vi "03 LV - Staged create-verify-staged update-archive.vi"   [LabVIEW 2020]
uses:
  client/Client/Client.lvclass
  client/AssetCreateStaging/AssetCreateStaging.lvclass
  client/Asset/Asset.lvclass
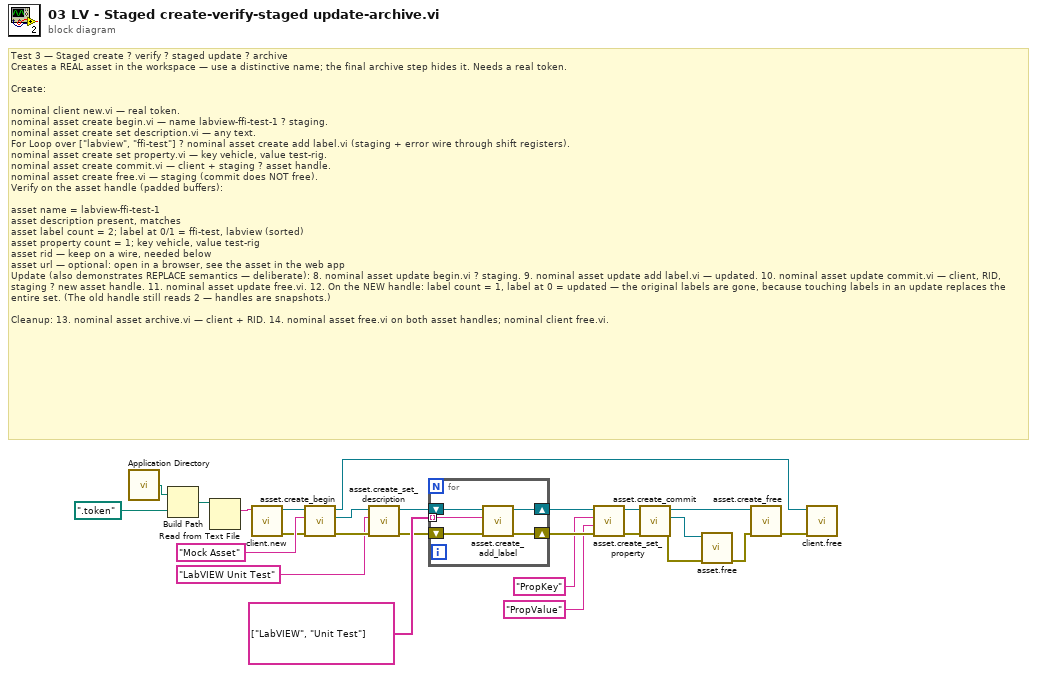
[diagram p0: block diagram]
diagram:
  # "Test 3 — Staged create ? verify ? staged update ? archive \nCreates a REAL asset in the workspace — use a distinctive name; the final archive step hides it. Needs a real token.\n\nCreate:\n\nnominal client new.vi — real token.\nnominal asset create begin.vi — name labview-ffi-test-1 ? staging.\nnominal asset create set description.vi — any text.\nFor Loop over [\"labview\", \"ffi-test\"] ? nominal asset create add label.vi (staging + error wire through shift registers).\nnominal asset create set property.vi — key vehicle, value test-rig.\nnominal asset create commit.vi — client + staging ? asset handle.\nnominal asset create free.vi — staging (commit does NOT free).\nVerify on the asset handle (padded buffers):\n\nasset name = labview-ffi-test-1\nasset description present, matches\nasset label count = 2; label at 0/1 = ffi-test, labview (sorted)\nasset property count = 1; key vehicle, value test-rig\nasset rid — keep on a wire, needed below\nasset url — optional: open in a browser, see the asset in the web app\nUpdate (also demonstrates REPLACE semantics — deliberate): 8. nominal asset update begin.vi ? staging. 9. nominal asset update add label.vi — updated. 10. nominal asset update commit.vi — client, RID, staging ? new asset handle. 11. nominal asset update free.vi. 12. On the NEW handle: label count = 1, label at 0 = updated — the original labels are gone, because touching labels in an update replaces the entire set. (The old handle still reads 2 — handles are snapshots.)\n\nCleanup: 13. nominal asset archive.vi — client + RID. 14. nominal asset free.vi on both asset handles; nominal client free.vi."
  n1 = call <vilib>:"Application Directory.vi"() -> ("Application Directory"=w24:path)
  n2 = Build Path(base path=w24, name or relative path=path ".token") -> (appended path=w22:path)
  n3 = Read from Text File(file (use dialog)=w22) -> (text=w21:string)  [unwired: 3 in, 3 out]
  n4 = call "client.new.vi"("token"=w21) -> ("error out"=w19:errorcluster, "Client out"=w13:refnum<class "Client.lvclass">)  [unwired: 9 in]
  n5 = call "asset.create_begin.vi"("error in"=w19, "name"="Mock Asset", "Client in"=w13) -> ("error out"=w17:errorcluster, "AssetCreateStaging"=w18:refnum<class "AssetCreateStaging.lvclass">, "Client out"=w12:refnum<class "Client.lvclass">)  [unwired: 6 in]
  n6 = call "asset.create_set_description.vi"("error in"=w17, "description"="LabVIEW Unit Test", "AssetCreateStaging in"=w18) -> ("error out"=w15:errorcluster, "AssetCreateStaging out"=w14:refnum<class "AssetCreateStaging.lvclass">)  [unwired: 7 in]
  n7 = for {
    shift-right: [w27] -> w10
    shift-left: w15 -> [w28]
    tunnel: string[] ["LabVIEW", "Unit Test"] ("label") -> [w30] mode=indexing
    shift-right: [w26] -> w11
    shift-left: w14 -> [w29]
    n8 = call "asset.create_add_label.vi"("error in"=w28, "label"=w30, "AssetCreateStaging in"=w29) -> ("error out"=w27:errorcluster, "AssetCreateStaging out"=w26:refnum<class "AssetCreateStaging.lvclass">)  [unwired: 7 in]
  }
  n9 = call "asset.create_set_property.vi"("error in"=w10, "value"="PropValue" ("key"), "key"="PropKey", "AssetCreateStaging in"=w11) -> ("error out"=w5:errorcluster, "AssetCreateStaging out"=w7:refnum<class "AssetCreateStaging.lvclass">)  [unwired: 6 in]
  n10 = call "asset.create_commit.vi"("error in"=w5, "AssetCreateStaging in"=w7) -> ("error out"=w3:errorcluster, "Asset out"=w4:refnum<class "Asset.lvclass">, "AssetCreateStaging out"=w6:refnum<class "AssetCreateStaging.lvclass">)  [unwired: 7 in]
  n11 = call "asset.free.vi"("error in"=w3, "asset in"=w4) -> ("error out"=w2:errorcluster)  [unwired: 9 in]
  n12 = call "asset.create_free.vi"("error in"=w2, "AssetCreateStaging in"=w6) -> ("error out"=w1:errorcluster)  [unwired: 9 in]
  n13 = call "client.free.vi"("error in"=w1, "Client in"=w12) -> ()  [unwired: 9 in, 1 out]
